vi "Init Actor Core.vi"(8 "error in (no error)":errorcluster, 11 "Measure Object in":refnum<class "Sequence Element.lvclass">) -> (0 "error out":errorcluster, 3 "Measure Object out":refnum<class "Sequence Element.lvclass">)   [LabVIEW 2016, in "Sequence Element.lvclass"]
uses:
  Sequence Element.lvclass
  Sequence Element.lvclass/Sequence Element.ctl
  Worker/Worker.lvclass
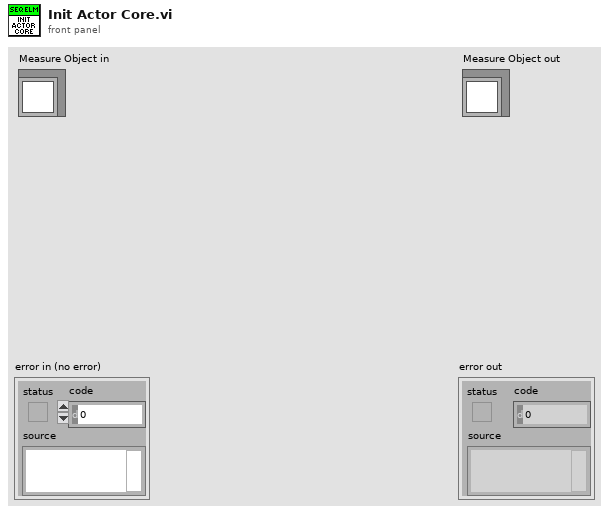
[diagram p1: front panel]
types:
  T1 = typedef "imagedata.ctl" = cluster{"image type":i32, "image depth":i32, "image":u8[], "mask":u8[], "colors":u32[], "Rectangle":cluster{"left":i16, "top":i16, "right":i16, "bottom":i16}}
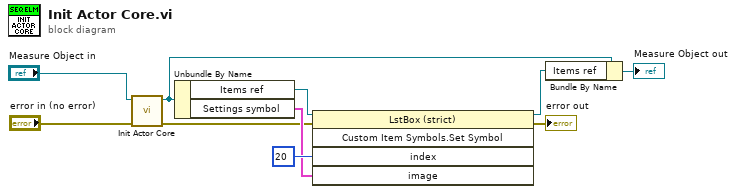
[diagram p0: block diagram]
diagram:
  n1 = call-parent "Init Actor Core.vi"("error in (no error)"="error in (no error)", "Measure Object in"="Measure Object in") -> ("error out"=w1:errorcluster, "Measure Object out"=w8:refnum<class "Sequence Element.lvclass">)  [unwired: 8 in]
  n2 = Unbundle By Name(w8) -> ("Items ref"=w7:refnum<vi>, "Settings symbol"=w5:T1)
  n3 = invoke class="LstBox (strict)" method="Custom Item Symbols.Set Symbol"(reference=w7, error in=w1, "index"=20 ("Index"), "image"=w5) -> (reference out=w3:refnum<vi>, error out=→"error out":errorcluster)  [unwired: 1 in, 3 out]
  n4 = Bundle By Name(cluster=w8, "Items ref"=w3) -> (→"Measure Object out":refnum<class "Sequence Element.lvclass">)
